vi "Data_Prod.vi"(7 "ProdType":enum16{"PC", "PI"}(ring), 8 "error in":errorcluster, 9 "cmd":string, 10 "SendCMD":bool, 11 "ReadOnlyIn":T1 {"CFG"."SystemResetTime" format="%<%H:%M:%S>t"}) -> (0 "error out":errorcluster, 2 "SendCMD":bool, 3 "ReadOnlyOut":T1 {"CFG"."SystemResetTime" format="%<%H:%M:%S>t"}, 4 "Stop":bool=TRUE)   [LabVIEW 2021, in "Main.lvlib"]
uses:
  Main.lvlib
  TypeDef/ReadOnly.ctl
  ValveCTRL/TypeDef/Queue_Cluster.ctl
  ValveCTRL/TypeDef/States_Enum.ctl
  ValveCTRL/TypeDef/CHs_List.ctl
  TypeDef/EventData.ctl
  <vilib>/MakerHub/LINX/Private/Type Defs/LINX Ref.ctl
  <vilib>/MakerHub/LINX/Private/Type Defs/Platform.ctl
  <vilib>/MakerHub/LINX/Private/Type Defs/Interface.ctl
  <vilib>/MakerHub/LINX/Private/Device/Type Defs/LINX Device Config.ctl
  <vilib>/MakerHub/LINX/Private/Device/Type Defs/TCP Config.ctl
  <vilib>/MakerHub/LINX/Private/Device/Type Defs/Channels.ctl
  Init/ReadInitCFG/TypeDef/CFG_Cluster.ctl
  <vilib>/ErrorRing/Error Ring.xnode
  ValveCTRL/ValveCTRL.lvlib
  UserEvent/UserEvent.lvlib
  <vilib>/Utility/error.llb/Error Cluster From Error Code.vi
  <vilib>/MakerHub/LINX/LMH-LINX.lvlib
  <vilib>/MakerHub/LINX/Private/Device/Device.lvlib
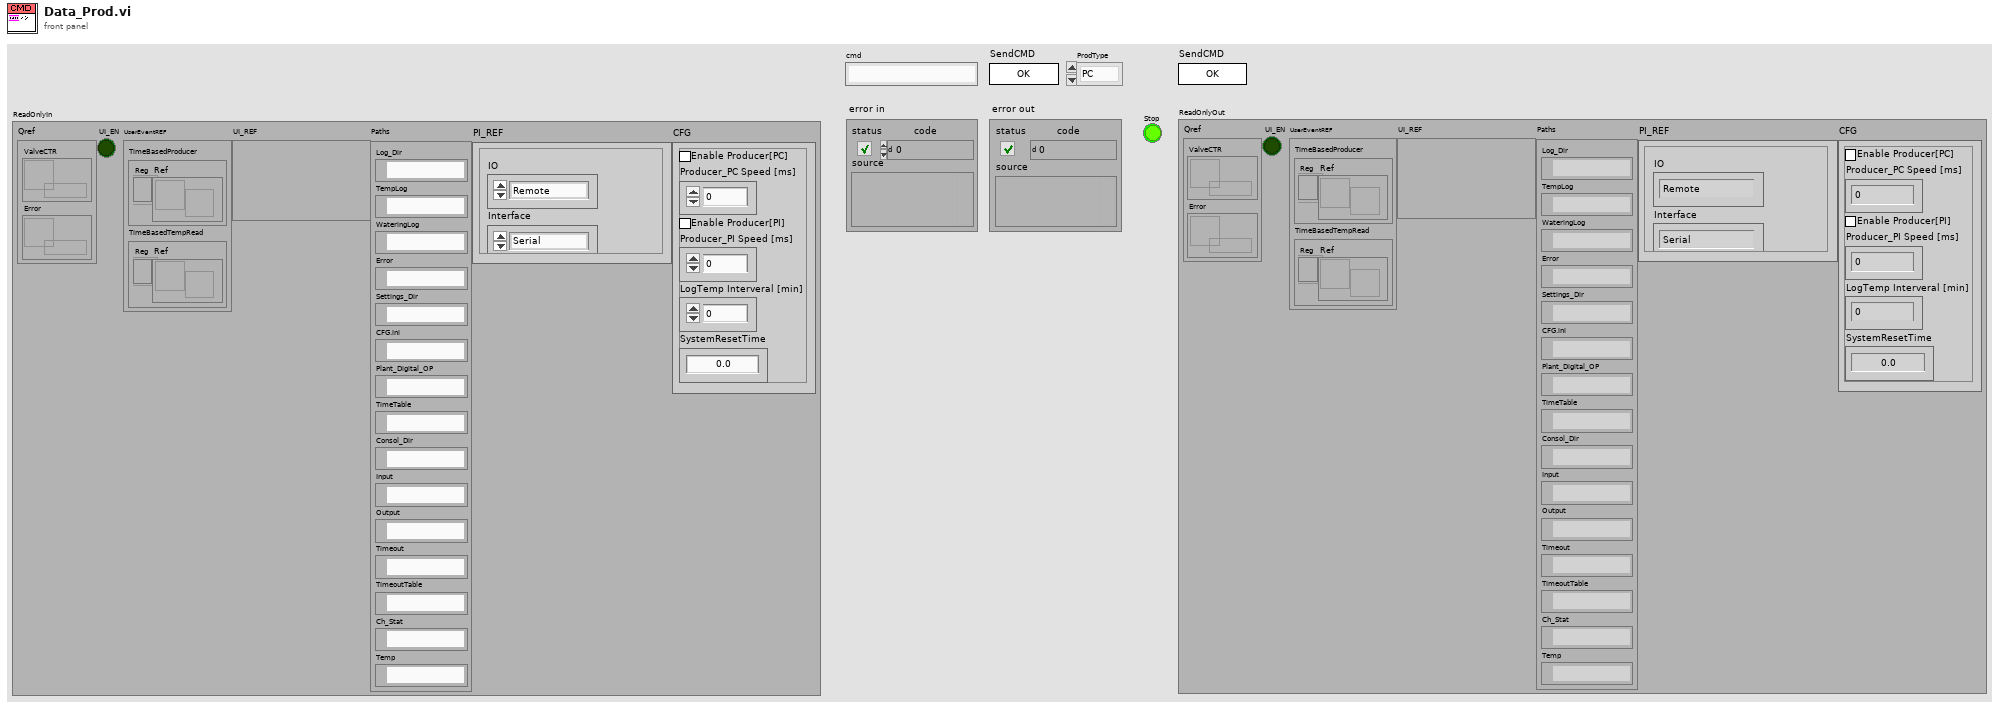
[diagram p1: front panel]
types:
  T1 = typedef "Main.lvlib/ReadOnly.ctl" = cluster{"Qref":cluster{"ValveCTR":refnum<queue>, "Error":refnum<queue>}, "UI_EN":bool, "UserEventREF":cluster{"TimeBasedProducer":cluster{"Reg":refnum<event-registration>, "Ref":refnum<user-event>}, "TimeBasedTempRead":cluster{"Reg":refnum<event-registration>, "Ref":refnum<user-event>}}, "UI_REF":variant, "Paths":cluster{"Log_Dir":path, "TempLog":path, "WateringLog":path, "Error":path, "Settings_Dir":path, "CFG.ini":path, "Plant_Digital_OP":path, "TimeTable":path, "Consol_Dir":path, "Input":path, "Output":path, "Timeout":path, "TimeoutTable":path, "Ch_Stat":path, "Temp":path}, "PI_REF":T2, "CFG":T8}
  T2 = typedef "LMH-LINX.lvlib/LINX Ref.ctl" = cluster{"IO":T3, "Interface":T4, "LINX Device Config":T5}
  T3 = typedef "LMH-LINX.lvlib/Platform.ctl" = enum16{"Remote", "Local"}
  T4 = typedef "LMH-LINX.lvlib/Interface.ctl" = enum16{"Serial", "TCP"}
  T5 = typedef "LMH-LINX.lvlib/Device.lvlib/LINX Device Config.ctl" = cluster{"Interface":T4, "COM Port":refnum<visa-resource-name>, "TCP Configuration":T6, "Device Family":u8, "Device ID":u8, "Device Name":string, "TCP Ref":refnum<k5>, "Channels":T7}
  T6 = typedef "LMH-LINX.lvlib/Device.lvlib/TCP Config.ctl" = cluster{"IP Address":string, "Port":u16}
  T7 = typedef "LMH-LINX.lvlib/Channels.ctl" = cluster{"DI":u8[], "DO":u8[], "AI":u8[], "AO":u8[], "PWM":u8[], "QE":u8[], "UART":u8[], "I2C 2":u8[], "SPI":u8[], "CAN":u8[], "Servo":u8[], "AI Ref (V)":dbl, "AI Resolution (Bits)":u8, "AO Ref (V)":dbl, "AO Resolution (Bits)":u8}
  T8 = typedef "Main.lvlib/CFG_Cluster.ctl" = cluster{"ProducerEn_PC":bool, "Producer_PC_ms":u32, "ProducerEn_PI":bool, "Producer_PI_ms":u32, "TempLogInterval":u32, "SystemResetTime":dbl}
  T9 = typedef "Main.lvlib/EventData.ctl" = cluster{"State":string, "Data":variant}
  T10 = typedef "ValveCTRL.lvlib/States_Enum.ctl" = enum16{"Open Pump", "Open Valve", "Wait Valve", "Close Pump", "Close Valve", "Save State", "StopLoop", "ValidCh"}
  T11 = typedef "ValveCTRL.lvlib/Queue_Cluster.ctl" = cluster{"State":T10, "Channel No":T12, "Duration[S]":dbl}
  T12 = typedef "ValveCTRL.lvlib/CHs_List.ctl" = u8
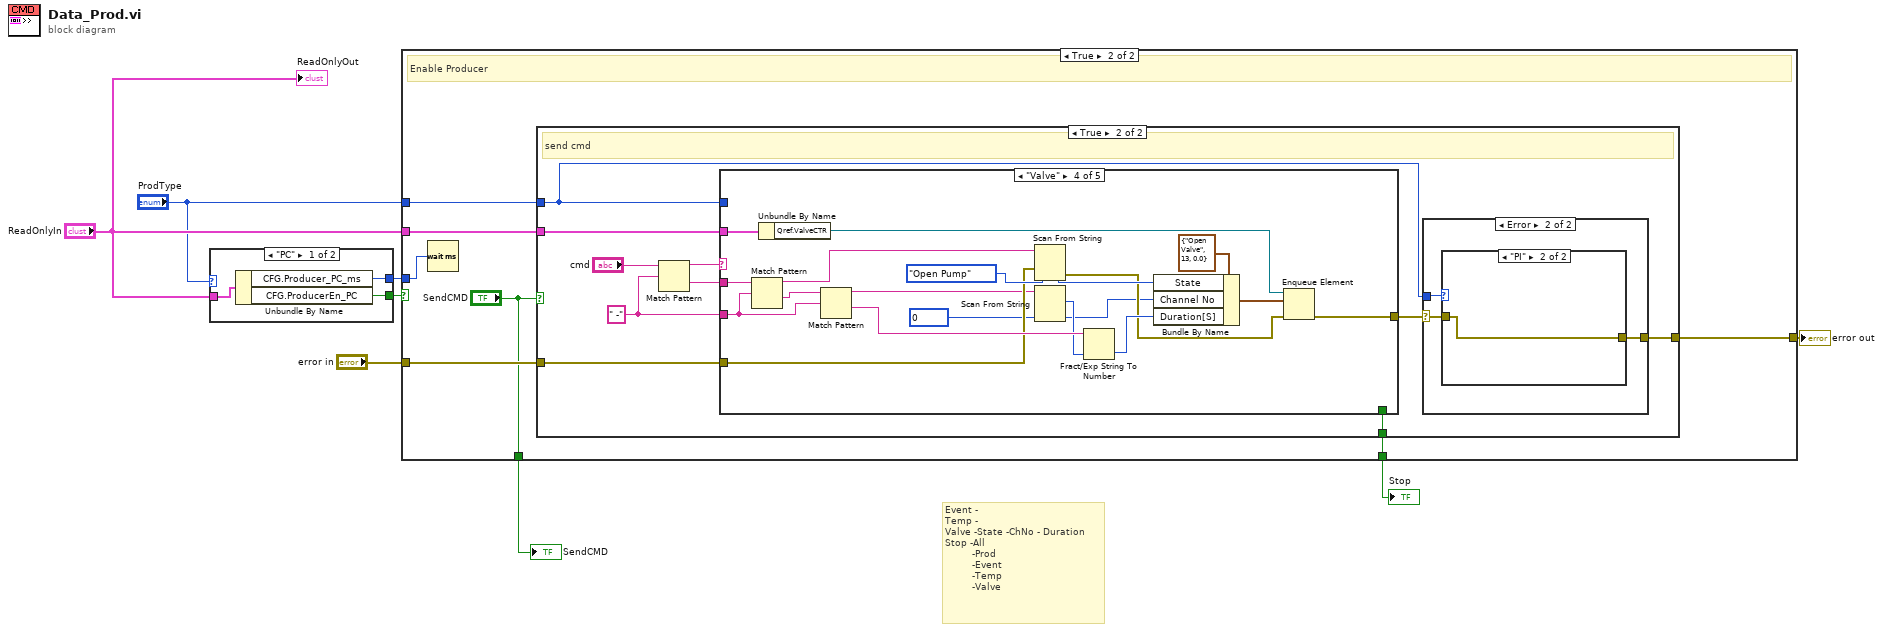
[diagram p0: block diagram]
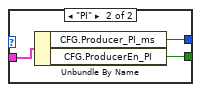
[diagram p2: hidden frame]
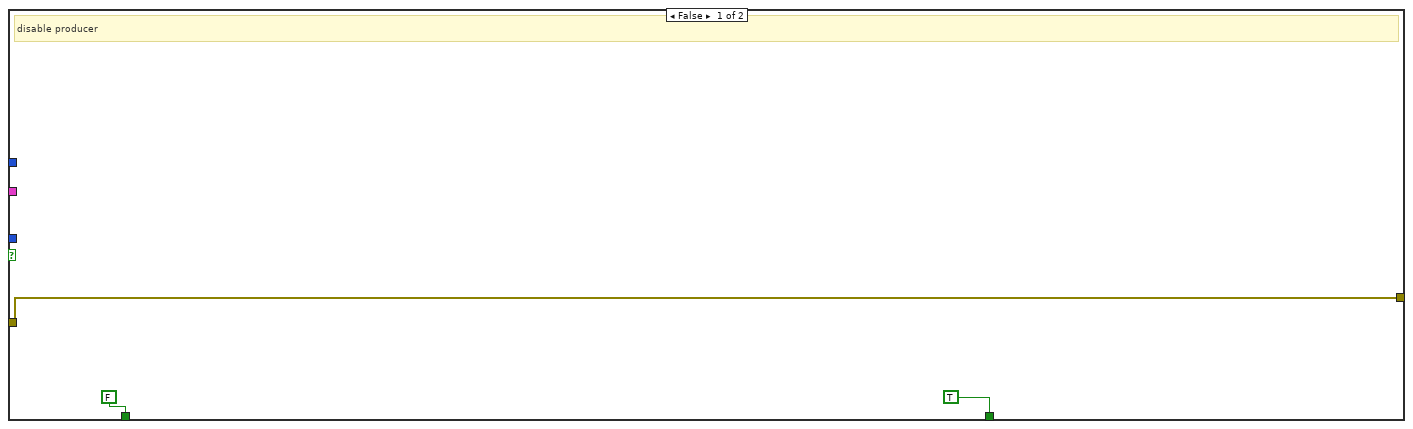
[diagram p3: hidden frame]
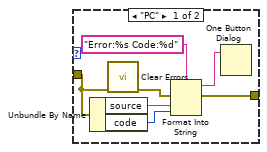
[diagram p6: hidden frame]
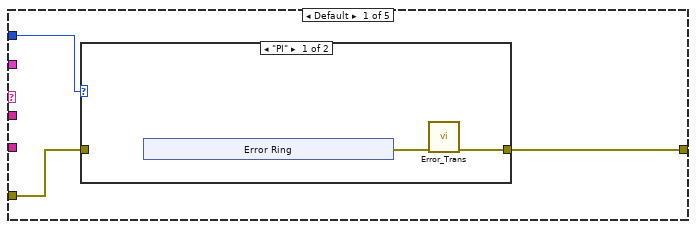
[diagram p7: hidden frame]
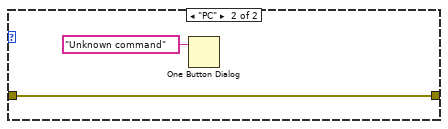
[diagram p8: hidden frame]
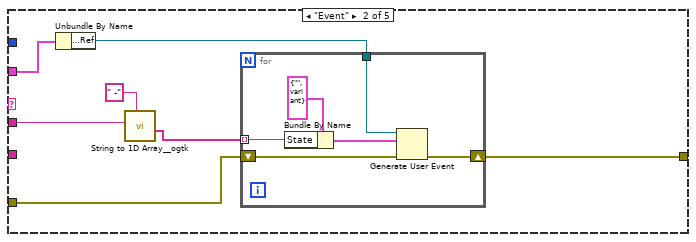
[diagram p9: hidden frame]
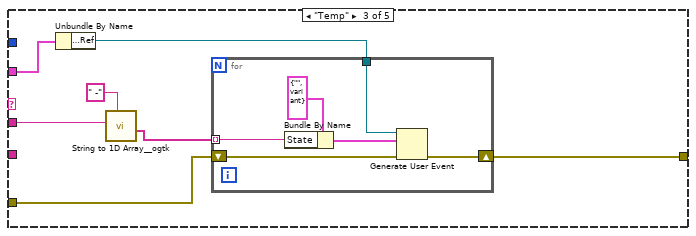
[diagram p10: hidden frame]
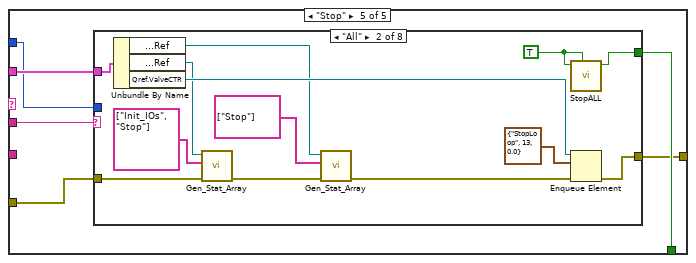
[diagram p11: hidden frame]
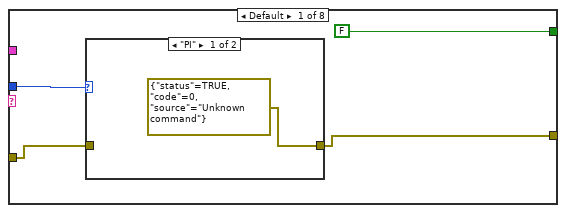
[diagram p12: hidden frame]
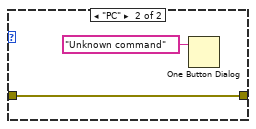
[diagram p13: hidden frame]
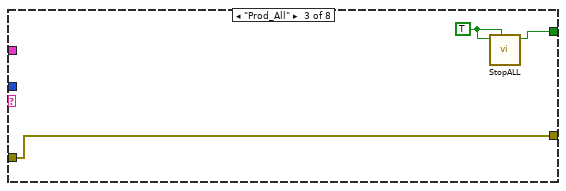
[diagram p14: hidden frame]
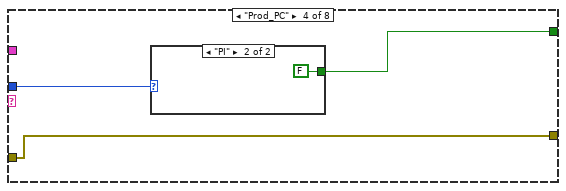
[diagram p15: hidden frame]
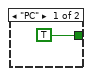
[diagram p16: hidden frame]
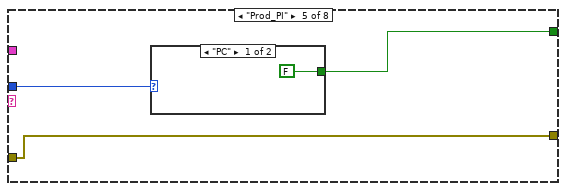
[diagram p17: hidden frame]
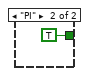
[diagram p18: hidden frame]
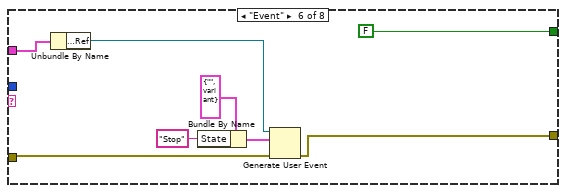
[diagram p19: hidden frame]
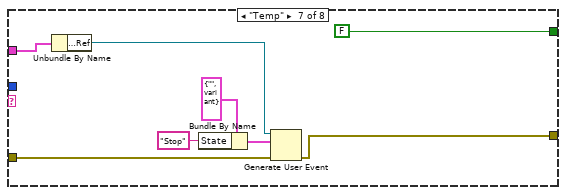
[diagram p20: hidden frame]
diagram:
  # "Event -\nTemp -\nValve -State -ChNo - Duration\nStop -All\n         -Prod\n         -Event\n         -Temp\n         -Valve"
  n1 = case shown="\"PC\"" "ProdType" {
    tunnel: "ReadOnlyIn" -> [w11 w14]
    tunnel: [w10 w13] -> w5
    tunnel: [w9 w12] -> w2
    frame "PC" {
      n2 = Unbundle By Name(w11) -> ("CFG.Producer_PC_ms"=w9:u32, "CFG.ProducerEn_PC"=w10:bool)
    }
    frame "PI" {
      n3 = Unbundle By Name(w14) -> ("CFG.Producer_PI_ms"=w12:u32, "CFG.ProducerEn_PI"=w13:bool)
    }
  }
  n4 = case shown="True" w5 {
    tunnel: "error in" -> [w16 w24]
    tunnel: [w16 w23] -> w7
    tunnel: "ReadOnlyIn" -> [_ w22]
    tunnel: [TRUE w21] -> w4
    tunnel: "ProdType" -> [_ w20]
    tunnel: w2 -> [_ w19]
    tunnel: [FALSE ("SendCMD") "SendCMD"] -> w1
    frame False {
      # "disable producer"
    }
    frame True {
      # "Enable Producer"
      n5 = Wait (ms)(milliseconds to wait=w19) -> ()  [unwired: 1 out]
      n6 = case shown="True" "SendCMD" {
        tunnel: w24 -> [w25 w33]
        tunnel: [w25 w30] -> w23
        tunnel: w22 -> [_ w29]
        tunnel: [_ w28] -> w21
        tunnel: w20 -> [_ w26]
        frame False {
          # "do not send cmd"
        }
        frame True {
          w35 = " -" ("search string/char (-)")
          # "send cmd"
          n7 = Match Pattern(string="cmd", regular expression=w35) -> (before substring=w34:string, after substring=w27:string)  [unwired: 1 in, 2 out]
          n8 = case shown="\"Valve\"" w34 {
            tunnel: w29 -> [_ w65 w78 w103 w107]
            tunnel: w27 -> [_ w61 w73 w99 w109]
            tunnel: w35 -> [_ _ _ w98 _]
            tunnel: w33 -> [w49 w63 w76 w90 w106]
            tunnel: [w48 w62 w75 w96 w105] -> w31
            tunnel: [_ _ _ _ w108] -> w28
            tunnel: w26 -> [w50 _ _ _ w104]
            frame Default {
              n9 = case shown="\"PI\"" w50 {
                tunnel: w49 -> [_ w57]
                tunnel: [w51 w57] -> w48
                frame "PI" {
                  n10 = xnode "Error Ring"() -> ("error out"=w52:errorcluster)
                  n11 = call "Error_Trans.vi"("Error In"=w52) -> ("Error Out"=w51:errorcluster)  [unwired: 9 in, 1 out]
                }
                frame "PC" {
                  n12 = One Button Dialog(message="Unknown command") -> ()  [unwired: 1 in, 1 out]
                }
              }
            }
            frame "Event" {
              n13 = Unbundle By Name(w65) -> ("UserEventREF.TimeBasedProducer.Ref"=w64:refnum<user-event>)
              n14 = call <userlib>:"String to 1D Array__ogtk.vi"("delimiter (Tab)"=" -", "string"=w61) -> ("Array of Strings"=w59:string[])  [unwired: 9 in]
              n15 = for {
                tunnel: w64 -> [w71]
                shift-right: [w67] -> w62
                shift-left: w63 -> [w68]
                tunnel: w59 -> [w66] mode=indexing
                n16 = Bundle By Name(cluster=T9 {"State"="", "Data"=variant} ("event data"), "State"=w66) -> (w69:T9)
                n17 = Generate User Event(user event=w71, event data cluster=w69, error in=w68) -> (error out=w67:errorcluster)  [unwired: 1 in, 1 out]
              }
            }
            frame "Temp" {
              n18 = Unbundle By Name(w78) -> ("UserEventREF.TimeBasedTempRead.Ref"=w77:refnum<user-event>)
              n19 = call <userlib>:"String to 1D Array__ogtk.vi"("delimiter (Tab)"=" -", "string"=w73) -> ("Array of Strings"=w72:string[])  [unwired: 9 in]
              n20 = for {
                tunnel: w77 -> [w84]
                shift-right: [w80] -> w75
                shift-left: w76 -> [w81]
                tunnel: w72 -> [w79] mode=indexing
                n21 = Bundle By Name(cluster=T9 {"State"="", "Data"=variant} ("event data"), "State"=w79) -> (w82:T9)
                n22 = Generate User Event(user event=w84, event data cluster=w82, error in=w81) -> (error out=w80:errorcluster)  [unwired: 1 in, 1 out]
              }
            }
            frame "Valve" {
              w87 = T12 0 items=["7"=7, "11"=11, "12"=12, "13"=13, "15"=15, "16"=16, "18"=18, "29"=29, "32"=32, "33"=33, "35"=35, "36"=36, "37"=37, "38"=38, "40"=40] ("Channel No")
              n23 = Match Pattern(string=w99, regular expression=w98) -> (before substring=w93:string, after substring=w95:string)  [unwired: 1 in, 2 out]
              n24 = Unbundle By Name(w103) -> ("Qref.ValveCTR"=w102:refnum<queue>)
              n25 = Match Pattern(string=w95, regular expression=w98) -> (before substring=w85:string, after substring=w94:string)  [unwired: 1 in, 2 out]
              n26 = Scan From String(input string=w93, error in=w90, default 1=States_Enum."Open Pump" ("State")) -> (error out=w89:errorcluster, output 1=w91:T10)  [unwired: 2 in, 2 out]
              n27 = Scan From String(input string=w85, default 1=w87) -> (offset past scan=w88:u32, output 1=w86:T12)  [unwired: 3 in, 2 out]
              n28 = Fract/Exp String To Number(string=w94, default (0 dbl)=w88) -> (number=w97:u32)  [unwired: 2 in, 1 out]
              n29 = Bundle By Name(cluster=T11 {"State"=enum."Open Valve", "Channel No"=13, "Duration[S]"=0.0} ("element"), "State"=w91, "Channel No"=w86, "Duration[S]"=w97) -> (w101:T11)
              n30 = Enqueue Element(queue=w102, element=w101, error in (no error)=w89) -> (error out=w96:errorcluster)  [unwired: 1 in, 2 out]
            }
            frame "Stop" {
              n31 = case shown="\"All\"" w109 {
                tunnel: [FALSE w123 w131 w133 w138 FALSE FALSE FALSE] -> w108
                tunnel: w107 -> [_ w129 _ _ _ w143 w152 w164]
                tunnel: w106 -> [w112 w128 w132 w135 w140 w145 w153 w161]
                tunnel: [w111 w127 w132 w135 w140 w144 w151 w163] -> w105
                tunnel: w104 -> [w110 _ _ w134 w139 _ _ _]
                frame Default {
                  n32 = case shown="\"PI\"" w110 {
                    tunnel: w112 -> [_ w115]
                    tunnel: [errorcluster {"status"=TRUE, "code"=0, "source"="Unknown command"} ("error in") w115] -> w111
                    frame "PI" {
                    }
                    frame "PC" {
                      n33 = One Button Dialog(message="Unknown command") -> ()  [unwired: 1 in, 1 out]
                    }
                  }
                }
                frame "All" {
                  w124 = TRUE
                  n34 = Unbundle By Name(w129) -> ("UserEventREF.TimeBasedTempRead.Ref"=w117:refnum<user-event>, "UserEventREF.TimeBasedProducer.Ref"=w121:refnum<user-event>, "Qref.ValveCTR"=w126:refnum<queue>)
                  n35 = call "Gen_Stat_Array.vi"("error in (no error)"=w128, "Array"=string[] ["Init_IOs", "Stop"], "User Event in"=w121) -> ("error out"=w120:errorcluster)  [unwired: 7 in, 1 out]
                  n36 = call "Gen_Stat_Array.vi"("error in (no error)"=w120, "Array"=string[] ["Stop"], "User Event in"=w117) -> ("error out"=w119:errorcluster)  [unwired: 7 in, 1 out]
                  n37 = call "StopALL.vi"("Write[F]"=w124, "StopIN"=w124) -> ("StopOUT"=w123:bool)  [unwired: 9 in]
                  n38 = Enqueue Element(queue=w126, element=T11 {"State"=enum."StopLoop", "Channel No"=13, "Duration[S]"=0.0}, error in (no error)=w119) -> (error out=w127:errorcluster)  [unwired: 1 in, 2 out]
                }
                frame "Prod_All" {
                  w130 = TRUE
                  n39 = call "StopALL.vi"("Write[F]"=w130, "StopIN"=w130) -> ("StopOUT"=w131:bool)  [unwired: 9 in]
                }
                frame "Prod_PC" {
                  n40 = case shown="\"PI\"" w134 {
                    tunnel: [TRUE FALSE] -> w133
                    frame "PC" {
                    }
                    frame "PI" {
                    }
                  }
                }
                frame "Prod_PI" {
                  n41 = case shown="\"PC\"" w139 {
                    tunnel: [FALSE TRUE] -> w138
                    frame "PC" {
                    }
                    frame "PI" {
                    }
                  }
                }
                frame "Event" {
                  n42 = Unbundle By Name(w143) -> ("UserEventREF.TimeBasedProducer.Ref"=w149:refnum<user-event>)
                  n43 = Bundle By Name(cluster=T9 {"State"="", "Data"=variant} ("event data"), "State"="Stop") -> (w147:T9)
                  n44 = Generate User Event(user event=w149, event data cluster=w147, error in=w145) -> (error out=w144:errorcluster)  [unwired: 1 in, 1 out]
                }
                frame "Temp" {
                  n45 = Unbundle By Name(w152) -> ("UserEventREF.TimeBasedTempRead.Ref"=w157:refnum<user-event>)
                  n46 = Bundle By Name(cluster=T9 {"State"="", "Data"=variant} ("event data"), "State"="Stop") -> (w155:T9)
                  n47 = Generate User Event(user event=w157, event data cluster=w155, error in=w153) -> (error out=w151:errorcluster)  [unwired: 1 in, 1 out]
                }
                frame "Valve" {
                  n48 = Unbundle By Name(w164) -> ("Qref.ValveCTR"=w166:refnum<queue>, "UserEventREF.TimeBasedProducer.Ref"=w159:refnum<user-event>)
                  n49 = call "Gen_Stat_Array.vi"("error in (no error)"=w161, "Array"=string[] ["Init_IOs"], "User Event in"=w159) -> ("error out"=w160:errorcluster)  [unwired: 7 in, 1 out]
                  n50 = Enqueue Element(queue=w166, element=T11 {"State"=enum."StopLoop", "Channel No"=13, "Duration[S]"=0.0}, error in (no error)=w160) -> (error out=w163:errorcluster)  [unwired: 1 in, 2 out]
                }
              }
            }
          }
          n51 = case shown="Error" w31 {
            selector: w31 -> [w36 w39]
            tunnel: [w36 w38] -> w30
            tunnel: w26 -> [_ w37]
            frame No Error {
            }
            frame Error {
              n52 = case shown="\"PI\"" w37 {
                tunnel: w39 -> [w43 w47]
                tunnel: [w40 w47] -> w38
                frame "PC" {
                  n53 = Unbundle By Name(w43) -> ("source"=w45:string, "code"=w44:i32)
                  n54 = call <vilib>:"Clear Errors.vi"("error in (no error)"=w43) -> ("error out"=w42:errorcluster)  [unwired: 5 in, 1 out]
                  n55 = Format Into String(format string="Error:%s Code:%d", error in=w42, w45, w44) -> (resulting string=w41:string, error out=w40:errorcluster)  [unwired: 1 in]
                  n56 = One Button Dialog(message=w41) -> ()  [unwired: 1 in, 1 out]
                }
                frame "PI" {
                }
              }
            }
          }
        }
      }
    }
  }
  "error out" <- w7
  "Stop" <- w4
  "SendCMD" <- w1
  "ReadOnlyOut" <- "ReadOnlyIn"
